vi "PIO Read U32 vs Byte-Swapped U32.vi"() -> ()   [LabVIEW 2016]
uses:
  <vilib>/Platform/TimedLoop/XDataNode/timing_clust.ctl
  <vilib>/Platform/TimedLoop/XDataNode/nitl_modes.ctl
  <vilib>/Platform/TimedLoop/XDataNode/wakeup.ctl
  Source/GE 5565PIORC/GE 5565PIORC Old.lvclass/GE 5565PIORC Old.ctl
  Source/GE 5565PIORC/VIs/Registers/Local Configuration.LAS1RR.Address Range.Get.vi
  Source/GE 5565PIORC/VIs/PIO/SubVIs/Change Endianness (U32).vi
  Source/GE 5565PIORC/VIs/Registers/Local Configuration.Get Register Offset.vi
  Source/GE 5565PIORC/GE 5565PIORC Old.lvclass
  <vilib>/platform/TimedLoop/XDataNode/XDataNode.xnode
  <vilib>/Platform/TimedLoop/XDataNode/XDNodeRunTimeDep.lvlib
panel:
  out "Byte-reversed U8 Array":u8[](array[numeric])
  out "U32 Array":u32[](array[numeric])
  in  "U32 Count":u32=100
  out "U32 Duration":dbl
  out "U32 Swapped Duration":dbl
  in  "VISA resource name":refnum<visa-resource-name>
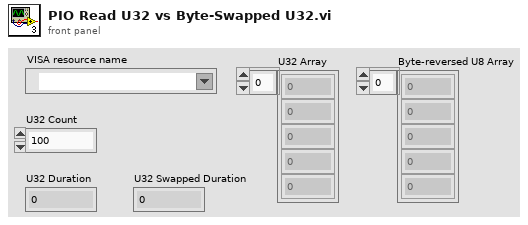
[diagram p1: front panel]
types:
  T1 = typedef "XDNodeRunTimeDep.lvlib/timing_clust.ctl" = cluster{"Expected End [f-1]":u64, "Actual End [f-1]":u64, "Finished Late? [f-1]":bool, "Expected End [i-1]":u64, "Actual End [i-1]":u64, "Finished Late? [i-1]":bool, "Expected Start [i]":u64, "Actual Start [i]":u64, "Expected Start [f]":u64, "Actual Start [f]":u64, "Source Name":string, "Structure Name":string, "Period":i64, "Deadline":i64, "Offset":i64, "Start":i64, "Priority":i32, "Timeout":i32, "Mode":T2, "Wakeup Reason":T3, "Error":errorcluster, "Source Type":string, "Secondary Source Type":string, "Global End Time":u64, "Global Start Time":u64, "Frame Duration":u64, "Iteration Duration":u64, "Assigned CPU":i32, "I/O Scan Engine Mode":u32}
  T2 = typedef "XDNodeRunTimeDep.lvlib/nitl_modes.ctl" = enum32{"No Change", "Process missed periods, maintain original phase", "Discard missed periods, maintain original phase", "Process missed periods, ignore original phase", "Discard missed periods, ignore original phase"}
  T3 = typedef "XDNodeRunTimeDep.lvlib/wakeup.ctl" = enum32{"Normal", "Aborted", "Asynchronous wakeup", "Timing source error", "Timed loop error", "Timeout"}
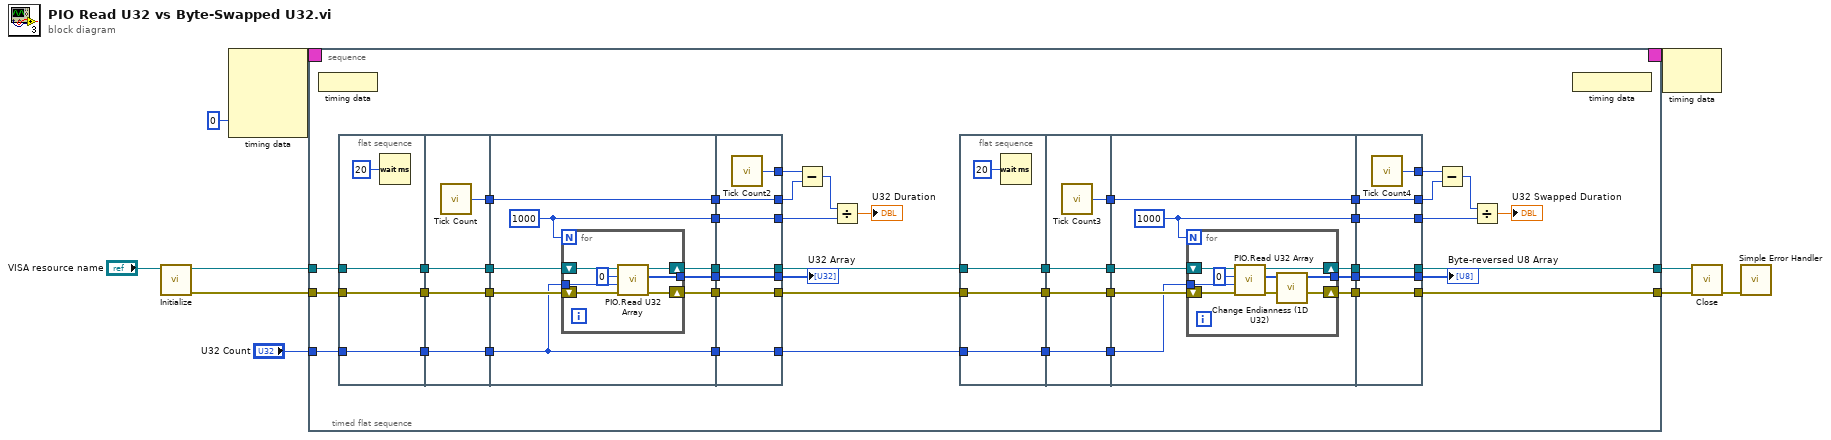
[diagram p0: block diagram]
diagram:
  n1 = call "Initialize.vi"("VISA resource name"="VISA resource name") -> ("error out"=w4:errorcluster, "GE 5565PIORC"=w5:refnum<class "GE 5565PIORC Old.lvclass">)  [unwired: 9 in]
  n2 = node-c288(0 ("Processor")) -> (w10:T1)  [unwired: 3 in]
  n3 = timed-sequence {
    timing: w10 -> [_]
    timing-out: [_] -> w9
    tunnel: w5 -> [w15]
    tunnel: w4 -> [w14]
    tunnel: [w13] -> w2
    tunnel: [w12] -> w3
    tunnel: "U32 Count" -> [w11]
    n4 = timed-flat-sequence {
      tunnel: w15 -> [w56]
      tunnel: w14 -> [w55]
      tunnel: [w33] -> w13
      tunnel: [w27] -> w12
      tunnel: w11 -> [w22]
      n5 = node-c288() -> ()  [unwired: 1 in]
      n6 = flat-sequence {
        tunnel: w56 -> [w93]
        tunnel: w55 -> [w92]
        tunnel: [w93] -> w53
        tunnel: [w92] -> w51
        tunnel: w22 -> [w91]
        tunnel: [w91] -> w21
        tunnel: [w98] -> w60
        tunnel: [w97] -> w54
        tunnel: w53 -> [w97]
        tunnel: [w96] -> w52
        tunnel: w51 -> [w96]
        tunnel: w21 -> [w95]
        tunnel: [w95] -> w20
        tunnel: w60 -> [w106]
        tunnel: [w106] -> w59
        tunnel: w54 -> [w102]
        tunnel: w52 -> [w103]
        tunnel: [w105] -> w50
        tunnel: [w104] -> w49
        tunnel: [w101] -> w32
        tunnel: [w100] -> w26
        tunnel: w20 -> [w99]
        tunnel: [w99] -> w19
        tunnel: [w120] -> w58
        tunnel: [w119] -> w57
        tunnel: w59 -> [w119]
        tunnel: w50 -> [w118]
        tunnel: [w118] -> w34
        tunnel: w49 -> [w117]
        tunnel: [w117] -> w47
        tunnel: w32 -> [w116]
        tunnel: [w116] -> w31
        tunnel: w26 -> [w115]
        tunnel: [w115] -> w24
        tunnel: w19 -> [w114]
        tunnel: [w114] -> w18
        frame #0 {
          n7 = Wait (ms)(milliseconds to wait=u32 20) -> ()  [unwired: 1 out]
        }
        frame #1 {
          n8 = call "Tick Count"() -> ("Tick Count(uSec)"=w98:u32)
        }
        frame #2 {
          w104 = 1000
          n9 = for {
            N: w104 -> [_]
            shift-right: [w111] -> w101
            shift-left: w102 -> [w113]
            shift-right: [w110] -> w105
            shift-left: w103 -> [w112]
            tunnel: [w108] -> w100
            tunnel: w99 -> [w107]
            n10 = call "PIO.Read U32 Array.vi"("error in (no error)"=w112, "count"=w107, "offset"=u32 0, "GE 5565PIORC in"=w113) -> ("error out"=w110:errorcluster, "values"=w108:u32[], "GE 5565PIORC out"=w111:refnum<class "GE 5565PIORC Old.lvclass">)  [unwired: 5 in]
          }
        }
        frame #3 {
          n11 = call "Tick Count2"() -> ("Tick Count(uSec)"=w120:u32)
        }
      }
      n12 = Subtract(x=w58, y=w57) -> (x-y=w48:u32)
      n13 = Divide(x=w48, y=w47) -> (x/y=→"U32 Duration":dbl)
      n14 = flat-sequence {
        tunnel: w34 -> [w63]
        tunnel: [w63] -> w45
        tunnel: w31 -> [w62]
        tunnel: [w62] -> w29
        tunnel: w18 -> [w61]
        tunnel: [w61] -> w16
        tunnel: [w68] -> w44
        tunnel: [w67] -> w43
        tunnel: w45 -> [w67]
        tunnel: [w66] -> w30
        tunnel: w29 -> [w66]
        tunnel: [w65] -> w17
        tunnel: w16 -> [w65]
        tunnel: w44 -> [w76]
        tunnel: [w76] -> w42
        tunnel: w43 -> [w73]
        tunnel: [w75] -> w41
        tunnel: [w74] -> w40
        tunnel: w30 -> [w72]
        tunnel: [w71] -> w28
        tunnel: [w70] -> w25
        tunnel: w17 -> [w69]
        tunnel: [w90] -> w39
        tunnel: [w89] -> w38
        tunnel: w42 -> [w89]
        tunnel: w41 -> [w88]
        tunnel: [w88] -> w33
        tunnel: w40 -> [w87]
        tunnel: [w87] -> w36
        tunnel: w28 -> [w86]
        tunnel: [w86] -> w27
        tunnel: w25 -> [w85]
        tunnel: [w85] -> w23
        frame #0 {
          n15 = Wait (ms)(milliseconds to wait=u32 20) -> ()  [unwired: 1 out]
        }
        frame #1 {
          n16 = call "Tick Count3"() -> ("Tick Count(uSec)"=w68:u32)
        }
        frame #2 {
          w74 = 1000
          n17 = for {
            N: w74 -> [_]
            shift-right: [w82] -> w75
            shift-left: w73 -> [w81]
            shift-right: [w83] -> w71
            shift-left: w72 -> [w84]
            tunnel: [w78] -> w70
            tunnel: w69 -> [w77]
            n18 = call "PIO.Read U32 Array.vi"("error in (no error)"=w81, "count"=w77, "offset"=u32 0, "GE 5565PIORC in"=w84) -> ("error out"=w82:errorcluster, "values"=w79:u32[], "GE 5565PIORC out"=w83:refnum<class "GE 5565PIORC Old.lvclass">)  [unwired: 5 in]
            n19 = call "Change Endianness (1D U32).vi"("array in"=w79) -> ("byte-reversed array out"=w78:u32[])  [unwired: 10 in]
          }
        }
        frame #3 {
          n20 = call "Tick Count4"() -> ("Tick Count(uSec)"=w90:u32)
        }
      }
      n21 = Subtract(x=w39, y=w38) -> (x-y=w37:u32)
      n22 = Divide(x=w37, y=w36) -> (x/y=→"U32 Swapped Duration":dbl)
      n23 = node-c288() -> ()  [unwired: 1 out]
      "U32 Array" <- w24
      "Byte-reversed U8 Array" <- w23
    }
  }
  n24 = node-c288(w9) -> ()  [unwired: 1 out]
  n25 = call "Close.vi"("error in (no error)"=w2, "GE 5565PIORC in"=w3) -> ("error out"=w7:errorcluster)  [unwired: 8 in, 1 out]
  n26 = call <vilib>:"Simple Error Handler.vi"("error in (no error)"=w7) -> ()  [unwired: 4 in, 5 out]
